vi "Create Facade.vi"(5 "SMOFacade in":refnum<class "SMOFacade.lvclass">, 6 "Filters":string[](array[string]), 8 "error in (no error)":errorcluster, 11 "SMO":refnum<class "SMO.lvclass">) -> (0 "error out":errorcluster, 3 "SMOFacade out":refnum<class "SMOFacade.lvclass">)   [LabVIEW 2013, in "SMOFacade.lvclass"]
uses:
  SMOFacade.lvclass
  SMO/SMO.lvclass
  SMOFacade.lvclass/SMOFacade.ctl
  Registry/Registry-SMO.lvclass
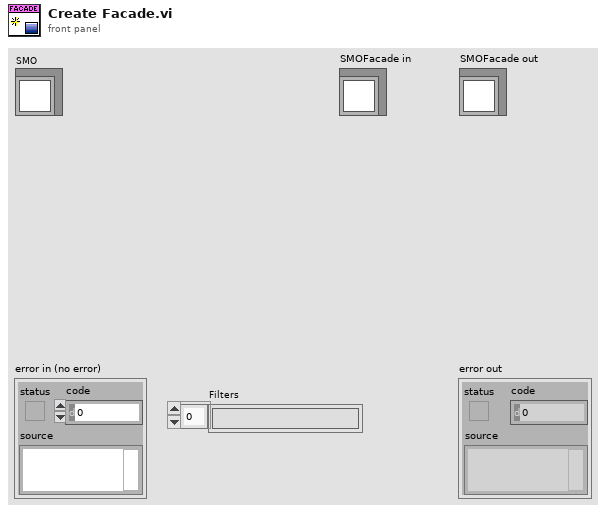
[diagram p1: front panel]
types:
  T1 = typedef "Registry-SMO.lvclass/SMO_API--Cluster.ctl" = cluster{"Method Name":string, "Full Method Name":string, "input string":string, "output string":string, "input type":variant, "output type":variant, "prototype":string, "Inputs":T2[], "Outputs":T2[]}
  T2 = typedef "Control Definition -- Cluster.ctl" = cluster{"Type Enum":T3, "Caption.Text":string, "DefVal":variant, "ControlIndex":i32, "Label.Text":string}
  T3 = typedef "VariantType.lvlib/Type.ctl" = enum8{"Invalid Type", "Void", "I8", "I16", "I32", "I64", "U8", "U16", "U32", "U64", "Single Float", "Double Float", "Extended Float", "Single Complex", "Double Complex", "Extended Complex", "Enum U8", "Enum U16", "Enum U32", "Enum U64", "Single Float With Unit", "Double Float With Unit", "Extended Float With Unit", "Single Complex with Unit", "Double Complex with Unit", "Extended Complex with Unit", "Boolean", "String", "Path", "Picture", "Tag", "Array", "Cluster", "Variant", "LV Variant", "Waveform", "Timestamp", "Digital Waveform", "Digital Data", "ExpressData", "Refnum", "External Data", "VI", "Poly VI", "LabVIEW Class Instance", "Fixed Point"}
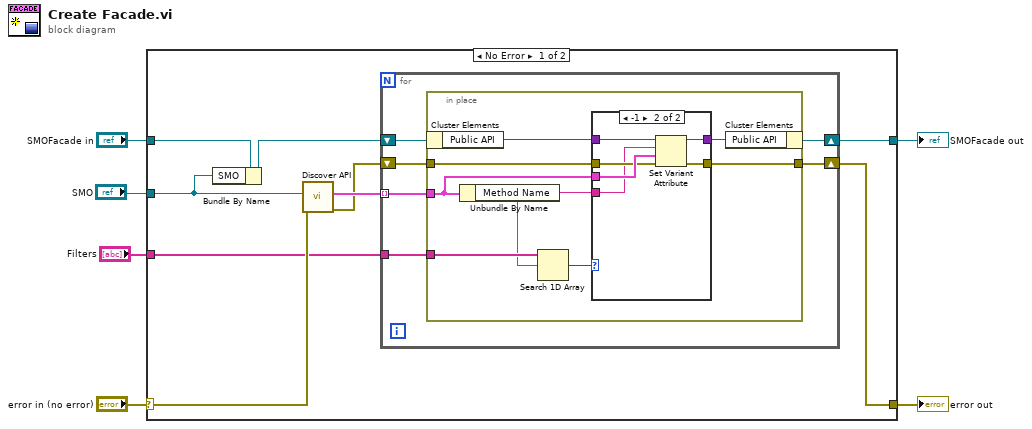
[diagram p0: block diagram]
diagram:
  n1 = case shown="No Error" "error in (no error)" {
    selector: "error in (no error)" -> [w13 w39]
    tunnel: [w8 w39] -> w5
    tunnel: [w11 w38] -> w3
    tunnel: "SMOFacade in" -> [w14 w38]
    tunnel: "SMO" -> [w15 _]
    tunnel: "Filters" -> [w7 _]
    frame No Error {
      n2 = Bundle By Name(cluster=w14, "SMO"=w15) -> (w12:refnum<class "SMOFacade.lvclass">)
      n3 = call "Discover API.vi"("error in (no error)"=w13, "SMO"=w15) -> ("error out"=w9:errorcluster, "PublicAPI"=w10:T1[])  [unwired: 8 in]
      n4 = for {
        shift-right: [w20] -> w11
        shift-left: w12 -> [w21]
        tunnel: w10 -> [w19] mode=indexing
        shift-right: [w17] -> w8
        shift-left: w9 -> [w18]
        tunnel: w7 -> [w16]
        n5 = in-place {
          in-place-border: w19 -> [w28]
          in-place-border: w18 -> [w26]
          in-place-border: [w25] -> w17
          in-place-border: w16 -> [w24]
          n6 = in-place-cluster #1(w21) -> ("Public API"=w29:variant)
          n7 = Unbundle By Name(w28) -> ("Method Name"=w23:string)
          n8 = Search 1D Array(1D array=w24, element=w23) -> (index of element=w22:i32)  [unwired: 1 in]
          n9 = case shown="-1" w22 {
            tunnel: w29 -> [w31 w37]
            tunnel: w28 -> [_ w36]
            tunnel: [w31 w35] -> w27
            tunnel: w26 -> [w30 w34]
            tunnel: [w30 w33] -> w25
            tunnel: w23 -> [_ w32]
            frame Default {
            }
            frame -1 {
              n10 = Set Variant Attribute(Variant=w37, name=w32, value=w36, error in=w34) -> (Variant out=w35:variant, error out=w33:errorcluster)  [unwired: 1 out]
            }
          }
          n11 = in-place-cluster #1("Public API"=w27) -> (w20:refnum<class "SMOFacade.lvclass">)
        }
      }
    }
    frame Error {
    }
  }
  "error out" <- w5
  "SMOFacade out" <- w3
